vi "Calibrate Photoresistor Theremin.vi"(3 "Error In":errorcluster, 4 "# Notes - 1 In":dbl, 6 "AI Task In":refnum<k21>) -> (0 "Error Out":errorcluster, 1 "V_PR Array":dbl[](array[numeric]), 2 "AI Task Out":refnum<k21>)   [LabVIEW 2020]
doc: "Calibrate Photoresistor Theremin.vi prompts the user for when they would like to record 7 different photoresistor voltages and outputs the logged voltages as an array."
uses:
  <vilib>/DAQmx/read.llb/DAQmx Read (Analog 1D DBL NChan 1Samp).vi
  <vilib>/DAQmx/miscellaneous.llb/DAQmx Fill In Error Info.vi
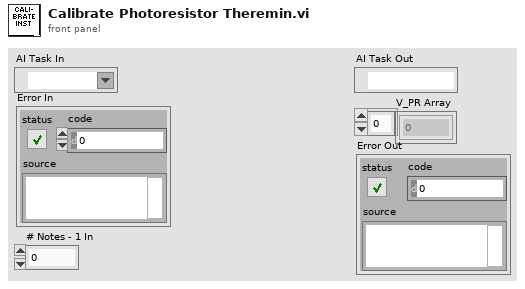
[diagram p1: front panel]
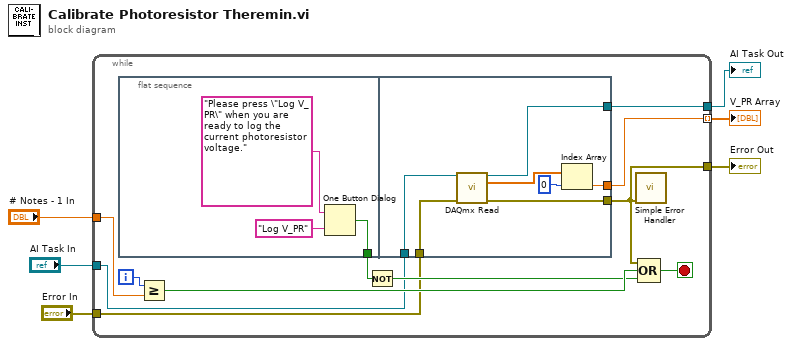
[diagram p0: block diagram]
diagram:
  n1 = while {
    tunnel: [w10] -> w2
    tunnel: "AI Task In" -> [w12]
    tunnel: [w11] -> w6
    tunnel: "Error In" -> [w9]
    tunnel: [w8] -> w3 mode=indexing
    tunnel: "# Notes - 1 In" -> [w7]
    i -> [w17]
    stop <- w16 stop-if-true
    n2 = flat-sequence {
      tunnel: [w18] -> w14
      tunnel: w12 -> [w27]
      tunnel: w9 -> [w26]
      tunnel: [w25] -> w11
      tunnel: [w24] -> w10
      tunnel: [w22] -> w8
      frame #0 {
        n3 = One Button Dialog(message="Please press \"Log V_PR\" when you are ready to log the current photoresistor voltage.", button name ("OK")="Log V_PR" ("T button name (\"OK\")")) -> (true=w18:bool)
      }
      frame #1 {
        n4 = call-poly <vilib>:"DAQmx Read.vi"("task/channels in"=w27, "error in"=w26) -> ("task out"=w25:refnum<k21>, "data"=w21:dbl[], "error out"=w24:errorcluster)  [unwired: 11 in]
        n5 = Index Array(array=w21, index=0) -> (element=w22:dbl)
      }
    }
    n6 = Greater Or Equal?(x=w17, y=w7) -> (x >= y?=w15:bool)
    n7 = Not(x=w14) -> (.not. x?=w13:bool)
    n8 = call <vilib>:"Simple Error Handler.vi"("error in (no error)"=w10) -> ()  [unwired: 4 in, 5 out]
    n9 = Compound Arithmetic op=OR(w10, w15, w13) -> (w16:bool)
  }
  "AI Task Out" <- w6
  "V_PR Array" <- w3
  "Error Out" <- w2
